vi "Basic Serial Write and Read1.vi"(4 "read":bool, 5 "write":bool, 6 "Close":bool, 8 "Open":bool, 9 "string to write":string="*IDN?\n", 11 "Setting":T1={"VISA resource name"="COM1", "baud rate"=57600, "data bits"=8, "parity"=0, "stop bits"=10, "flow control"=0, "Read TimeOut (ms)"=500, "Byte Read Count(999Exit)"=500, "Read End Str"=FALSE, "End String"="\r\n"} {"flow control" items=["None"=0, "XON/XOFF"=1, "RTS/CTS"=2, "DTR/DSR"=4]; "stop bits" items=["1.0"=10, "1.5"=15, "2.0"=20]; "parity" items=["None", "Odd", "Even", "Mark", "Space"]; "data bits" min=5 max=8 step=1}) -> (0 "bytes read":u32, 1 "read string":string, 3 "error out":errorcluster)   [LabVIEW 2024]
doc: "The Basic Serial Read and Write example performs a Serial Port Read, a Serial Port Write, or a combination of these actions. The user selects the actions (read or write) on the front panel. If both are selected, the VI will write the data first, read data, and then close the VISA session that is opened to the port. This VI will wait until the specified number of bytes is received at the port or until a termination character is read.\n\nINSTRUCTIONS:\n1) Select the serial resource and configuration parameters (baud rate, data bits, parity, stop bits, flow control).\n2) Select the operations to be performed. \n3) Connect the serial port to your device. If no device is available, perform a loopback test by doing one of the following. Short pins 2 and 3 on a RS-232 cable or short pin 4 to pin 8 and pin 5 to pin 9 on a RS-485/422 cable. \n4) Run the VI to see the data read. (The \"read string\" will match the \"string to write\" if a loopback test was performed.)\n\nNote: The parameters set for the serial port must match the parameters of the connected instrument or device. In this example, the bytes to read parameter specifies the number of bytes that the serial port reads. If there were more bytes at the port than the number specified in bytes to read, those bytes would not be read. Also, if you specify to read more bytes than the number of bytes actually read, you might receive a timeout error message.\n\nOn the block diagram, the Configure Serial Port VI sets the configuration parameters. The front panel displays the controls used to configure the basic parameters, such as baud rate, data bits, and parity. Constants configure the other parameters the user probably does not need set. After the VISA Configure Serial Port VI opens the VISA session and configures the port, the VI passes the VISA resource name to other VIs that perform operations on that VISA resource. The VISA Write function sends a command to the serial device and the VISA Read function returns data based on the command. The VISA Close function then closes the reference to the serial device. It is important to close the reference; otherwise communication through with that port through protocols other than VISA might not be possible."
uses:
  <vilib>/Utility/error.llb/DialogType.ctl
  <vilib>/Instr/_visa.llb/VISA Configure Serial Port (Instr).vi
panel:
  out "read buffer":string
  out "Tact Time":u32
  out "return count":u32
  # "On Windows/Linux, consider using the Instrument Driver Finder (Help>>Find Instrument Drivers) to search for an instrument driver for your instrument."
  # "Select the serial resource and the operations (Read, Write, or both) to be performed.  If both are selected, the VI will write the data first, read data and then close the VISA session that is opened to the port.  This VI will wait until the specified number of bytes is received at the port or until a termination character is read."
  # "For additional information select File >> VI Properties >> Documentation"
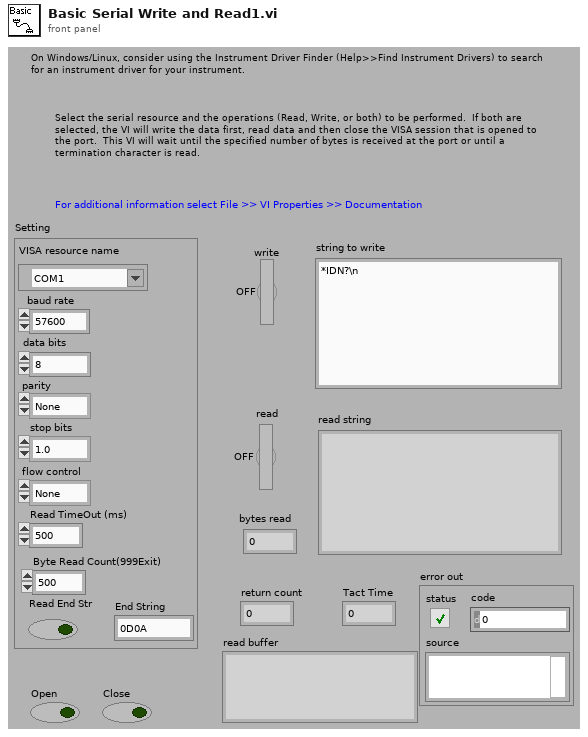
[diagram p1: front panel]
types:
  T1 = cluster{"VISA resource name":refnum<visa-resource-name>, "baud rate":u32, "data bits":u16, "parity":u16, "stop bits":u16, "flow control":u16, "Read TimeOut (ms)":u32, "Byte Read Count(999Exit)":u32, "Read End Str":bool, "End String":string}
  T2 = typedef "DialogType.ctl" = u16
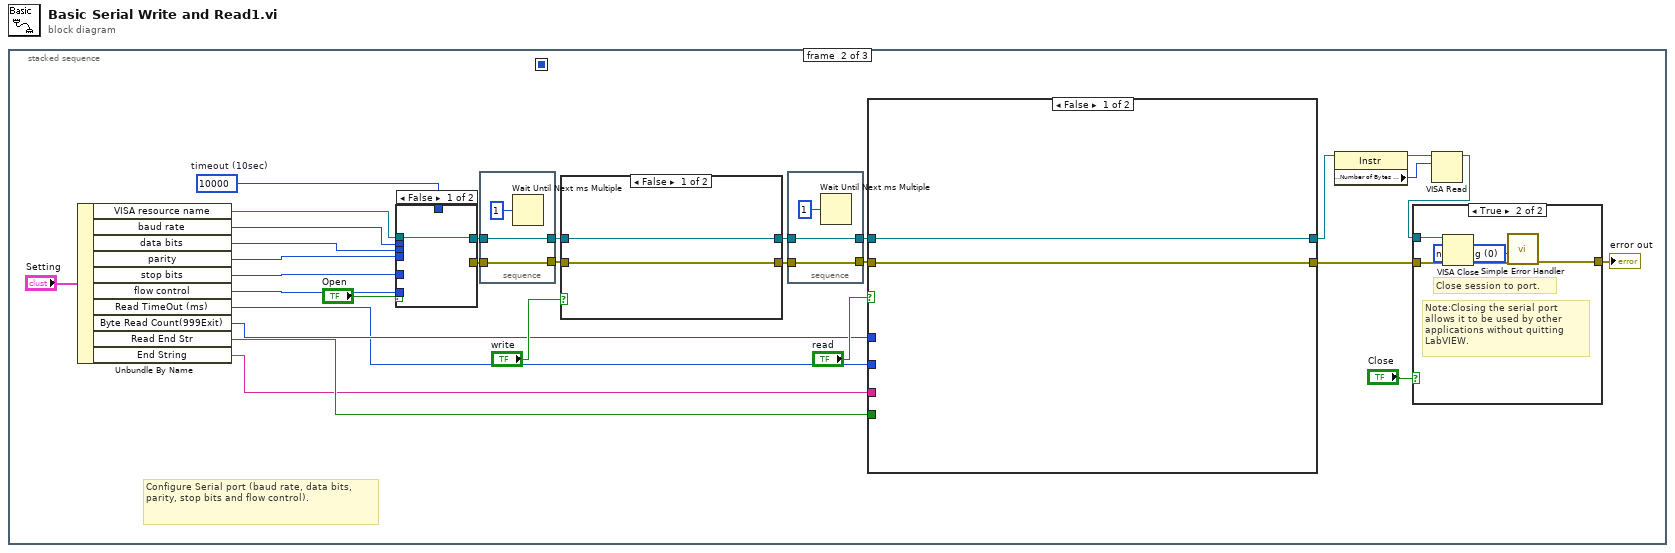
[diagram p0: block diagram]
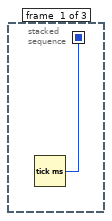
[diagram p2: hidden frame]
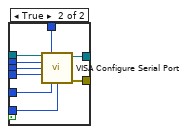
[diagram p4: hidden frame]
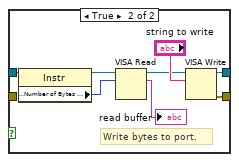
[diagram p5: hidden frame]
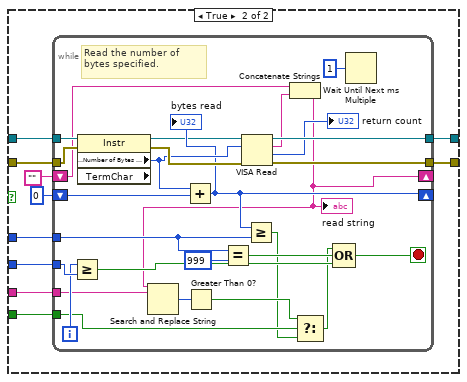
[diagram p6: hidden frame]
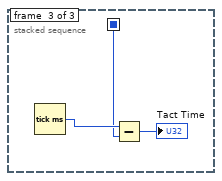
[diagram p7: hidden frame]
diagram:
  n1 = stacked-sequence {
    seq-local: [w1 _ _] -> [_ _ w103]
    frame #0 {
      n2 = Tick Count (ms)() -> (millisecond timer value=w1:u32)
    }
    frame #1 {
      w29 = u32 10000  # timeout (10sec)
      # "Configure Serial port (baud rate, data bits, parity, stop bits and flow control)."
      n3 = Unbundle By Name("Setting") -> ("VISA resource name"=w26:refnum<visa-resource-name>, "baud rate"=w25:u32, "data bits"=w24:u16, "parity"=w23:u16, "stop bits"=w22:u16, "flow control"=w21:u16, "Read TimeOut (ms)"=w19:u32, "Byte Read Count(999Exit)"=w20:u32, "Read End Str"=w18:bool, "End String"=w17:string)
      n4 = case shown="False" "Open" {
        tunnel: [_ w52] -> w8
        tunnel: [w43 w51] -> w10
        tunnel: w29 -> [_ w50]
        tunnel: w26 -> [w43 w49]
        tunnel: w25 -> [_ w48]
        tunnel: w24 -> [_ w47]
        tunnel: w23 -> [_ w46]
        tunnel: w22 -> [_ w45]
        tunnel: w21 -> [_ w44]
        frame False {
        }
        frame True {
          n5 = call-poly "VISA Configure Serial Port"("VISA resource name"=w49, "timeout (10sec)"=w50, "baud rate (9600)"=w48, "data bits (8)"=w47, "parity (0:none)"=w46, "stop bits (10: 1 bit)"=w45, "flow control (0:none)"=w44) -> ("VISA resource name out"=w51:refnum<visa-resource-name>, "error out"=w52:errorcluster)  [unwired: 2 in, 5 out]
        }
      }
      n6 = stacked-sequence {
        tunnel: w10 -> [w37]
        tunnel: [w37] -> w9
        tunnel: w8 -> [w36]
        tunnel: [w36] -> w7
        frame #0 {
          n7 = Wait Until Next ms Multiple(millisecond multiple=u32 1) -> ()  [unwired: 1 out]
        }
      }
      n8 = case shown="False" "write" {
        tunnel: [w53 w62] -> w5
        tunnel: w9 -> [w54 w59]
        tunnel: [w54 w60] -> w6
        tunnel: w7 -> [w53 _]
        frame False {
        }
        frame True {
          # "Write bytes to port."
          n9 = property class="Instr"(reference=w59) -> (reference out=w58:refnum<visa-resource-name>, "Serial Settings:Number of Bytes at Serial Port"=w57:u32)  [unwired: 1 in, 1 out]
          n10 = VISA Read(VISA resource name=w58, byte count=w57) -> (VISA resource name out=w56:refnum<visa-resource-name>, read buffer=→"read buffer":string)  [unwired: 1 in, 2 out]
          n11 = VISA Write(VISA resource name=w56, write buffer="string to write") -> (VISA resource name out=w60:refnum<visa-resource-name>, error out=w62:errorcluster)  [unwired: 1 in, 1 out]
        }
      }
      n12 = stacked-sequence {
        tunnel: w6 -> [w34]
        tunnel: [w34] -> w4
        tunnel: w5 -> [w33]
        tunnel: [w33] -> w3
        frame #0 {
          n13 = Wait Until Next ms Multiple(millisecond multiple=u32 1) -> ()  [unwired: 1 out]
        }
      }
      n14 = case shown="False" "read" {
        tunnel: w3 -> [w64 w67]
        tunnel: [w64 w65] -> w30
        tunnel: [w63 w66] -> w12
        tunnel: w4 -> [w63 w68]
        tunnel: w20 -> [_ w72]
        tunnel: w19 -> [_ w71]
        tunnel: w18 -> [_ w70]
        tunnel: w17 -> [_ w69]
        frame False {
        }
        frame True {
          n15 = while {
            tunnel: [w101] -> w65
            tunnel: [w100] -> w66
            tunnel: w68 -> [w99]
            tunnel: w67 -> [w98]
            shift-right: [w83] -> _
            shift-left: "" -> [w95]
            shift-right: [w91] -> _
            shift-left: u32 0 -> [w93]
            tunnel: w72 -> [w88]
            tunnel: w71 -> [w85]
            tunnel: w70 -> [w80]
            tunnel: w69 -> [w77]
            i -> [w84]
            stop <- w90 stop-if-true
            # "Read the number of bytes specified."
            n16 = Greater Or Equal?(x=w84, y=w85) -> (x >= y?=w86:bool)
            n17 = property class="Instr" props=["Serial Settings:Number of Bytes at Serial Port", "TermChar"](reference=w99, error in=w98) -> (reference out=w76:refnum<visa-resource-name>, error out=w97:errorcluster, "Serial Settings:Number of Bytes at Serial Port"=w92:u32)  [unwired: 1 out]
            n18 = Add(x=w92, y=w93) -> (x+y=w91:u32)
            "bytes read" <- w91
            n19 = Equal?(x=w88, y=u32 999) -> (x = y?=w89:bool)
            n20 = VISA Read(VISA resource name=w76, byte count=w92, error in (no error)=w97) -> (VISA resource name out=w100:refnum<visa-resource-name>, read buffer=w94:string, return count=→"return count":u32, error out=w101:errorcluster)
            n21 = Greater Or Equal?(x=w91, y=w88) -> (x >= y?=w78:bool)
            n22 = Concatenate Strings(w95, w94) -> (w83:string)
            "read string" <- w83
            n23 = Search and Replace String(input string=w83, search string=w77) -> (number of replacements=w82:i32)  [unwired: 6 in, 3 out]
            n24 = Greater Than 0?(x=w82) -> (x > 0?=w81:bool)
            n25 = Select(t=w81, s=w80, f=w78) -> (s? t:f=w79:bool)
            n26 = Compound Arithmetic op=OR(w79, w89, w86) -> (w90:bool)
            n27 = Wait Until Next ms Multiple(millisecond multiple=u32 1) -> ()  [unwired: 1 out]
          }
        }
      }
      n28 = property class="Instr"(reference=w12) -> (reference out=w13:refnum<visa-resource-name>, "Serial Settings:Number of Bytes at Serial Port"=w14:u32)  [unwired: 1 in, 1 out]
      n29 = VISA Read(VISA resource name=w13, byte count=w14) -> (VISA resource name out=w11:refnum<visa-resource-name>)  [unwired: 1 in, 3 out]
      n30 = case shown="True" "Close" {
        tunnel: w30 -> [_ w42]
        tunnel: w11 -> [_ w41]
        tunnel: [_ w39] -> w2
        frame False {
        }
        frame True {
          w38 = T2 0 items=["no dialog", "OK message", "continue or stop message", "OK message + warnings", "continue/stop + warnings"] ("type of dialog (OK msg:1)")
          # "Note:Closing the serial port allows it to be used by other applications without quitting LabVIEW."
          # "Close session to port."
          n31 = VISA Close(VISA resource name=w41, error in (no error)=w42) -> (error out=w40:errorcluster)
          n32 = call <vilib>:"Simple Error Handler.vi"("type of dialog (OK msg:1)"=w38, "error in (no error)"=w40) -> ("error out"=w39:errorcluster)  [unwired: 7 out]
        }
      }
      "error out" <- w2
    }
    frame #2 {
      n33 = Tick Count (ms)() -> (millisecond timer value=w104:u32)
      n34 = Subtract(x=w104, y=w103) -> (x-y=→"Tact Time":u32)
    }
  }
